vi "harmonics_2021a.vi"() -> ()   [LabVIEW 2024]
uses:
  <vilib>/Analysis/5stat.llb/RMS (DBL).vi
  <vilib>/Utility/file.llb/Read Delimited Spreadsheet (DBL).vi
  <vilib>/measure/matone.llb/Harmonic Distortion Analyzer 1 Chan.vi
  <vilib>/measure/matone.llb/Extract Multiple Tone Information 1 Chan.vi
  <vilib>/measure/NI_MAPro.lvlib
  <vilib>/Analysis/NI_AALPro.lvlib
panel:
  out "grafic energieni consumate":dbl[](graph)
  out "timp":dbl
  out "E [Ws]":dbl
  in  "file path (dialog if empty)":path=path "C:/Users/ciprian/OneDrive - Universitatea Politehnica Timisoara/DESKTOP-LAPTOP HOME 12.12.2021/GR 1 _ 2 _PS_2021.txt"
  in  "Nr_spire":dbl=5.0
  out "D [VAD]":dbl
  out "Q [VA]":dbl
  out "P [W]":dbl
  out "S [VA]":dbl
  out "rms value voltage":dbl format="%0.2f"
  out "rms current 3rd harmonic":dbl format="%0.2f"
  out "rms currnt fundamental":dbl format="%0.2f"
  out "3rd harmonic graph":waveform(dbl)(graph)
  out "3rd current harmonic signal":waveform(dbl)
  in  "export mode 2":T1(ring)=enum."harmonics only"
  in  "export mode":T1(ring)=enum."fundamental signal"
  out "fundamental signal":waveform(dbl)
  out "fundamental graph":waveform(dbl)(graph)
  out "multiple tone information":T2(array[cluster]) {"detected phase (deg)" format="%_6g"; "detected amplitude" format="%_6p"; "detected frequency" format="%_6p"}
  out "input signal graph":dbl[](graph)
  out "t          UMv       UMi           E":dbl[][](array[numeric])
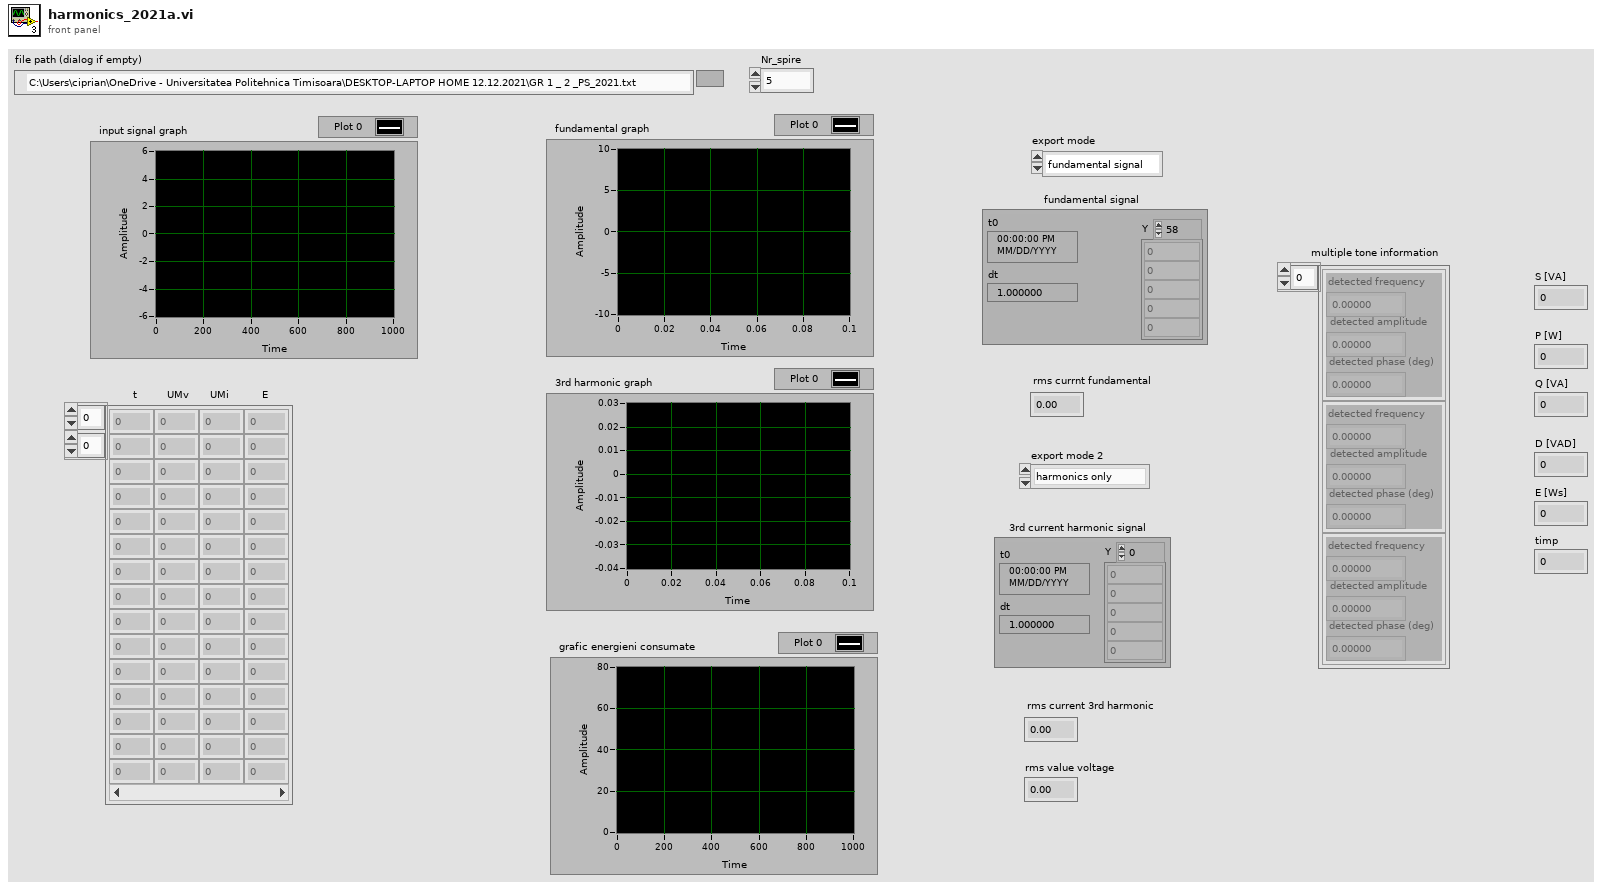
[diagram p1: front panel]
types:
  T1 = enum16{"none", "input signal", "fundamental signal", "residual signal", "harmonics only", "noise and spurs"}
  T2 = cluster{"detected frequency":dbl, "detected amplitude":dbl, "detected phase (deg)":dbl}[]
  T3 = enum32{"none", "input signal", "detected signal", "residual signal"}
  T4 = cluster{"exported time signal":waveform(dbl), "exported spectrum (dB)":cluster{"f0":dbl, "df":dbl, "dB Spectrum (Hann)":dbl[]}}
  T5 = cluster{"detected frequency":dbl, "detected amplitude":dbl, "detected phase (deg)":dbl}
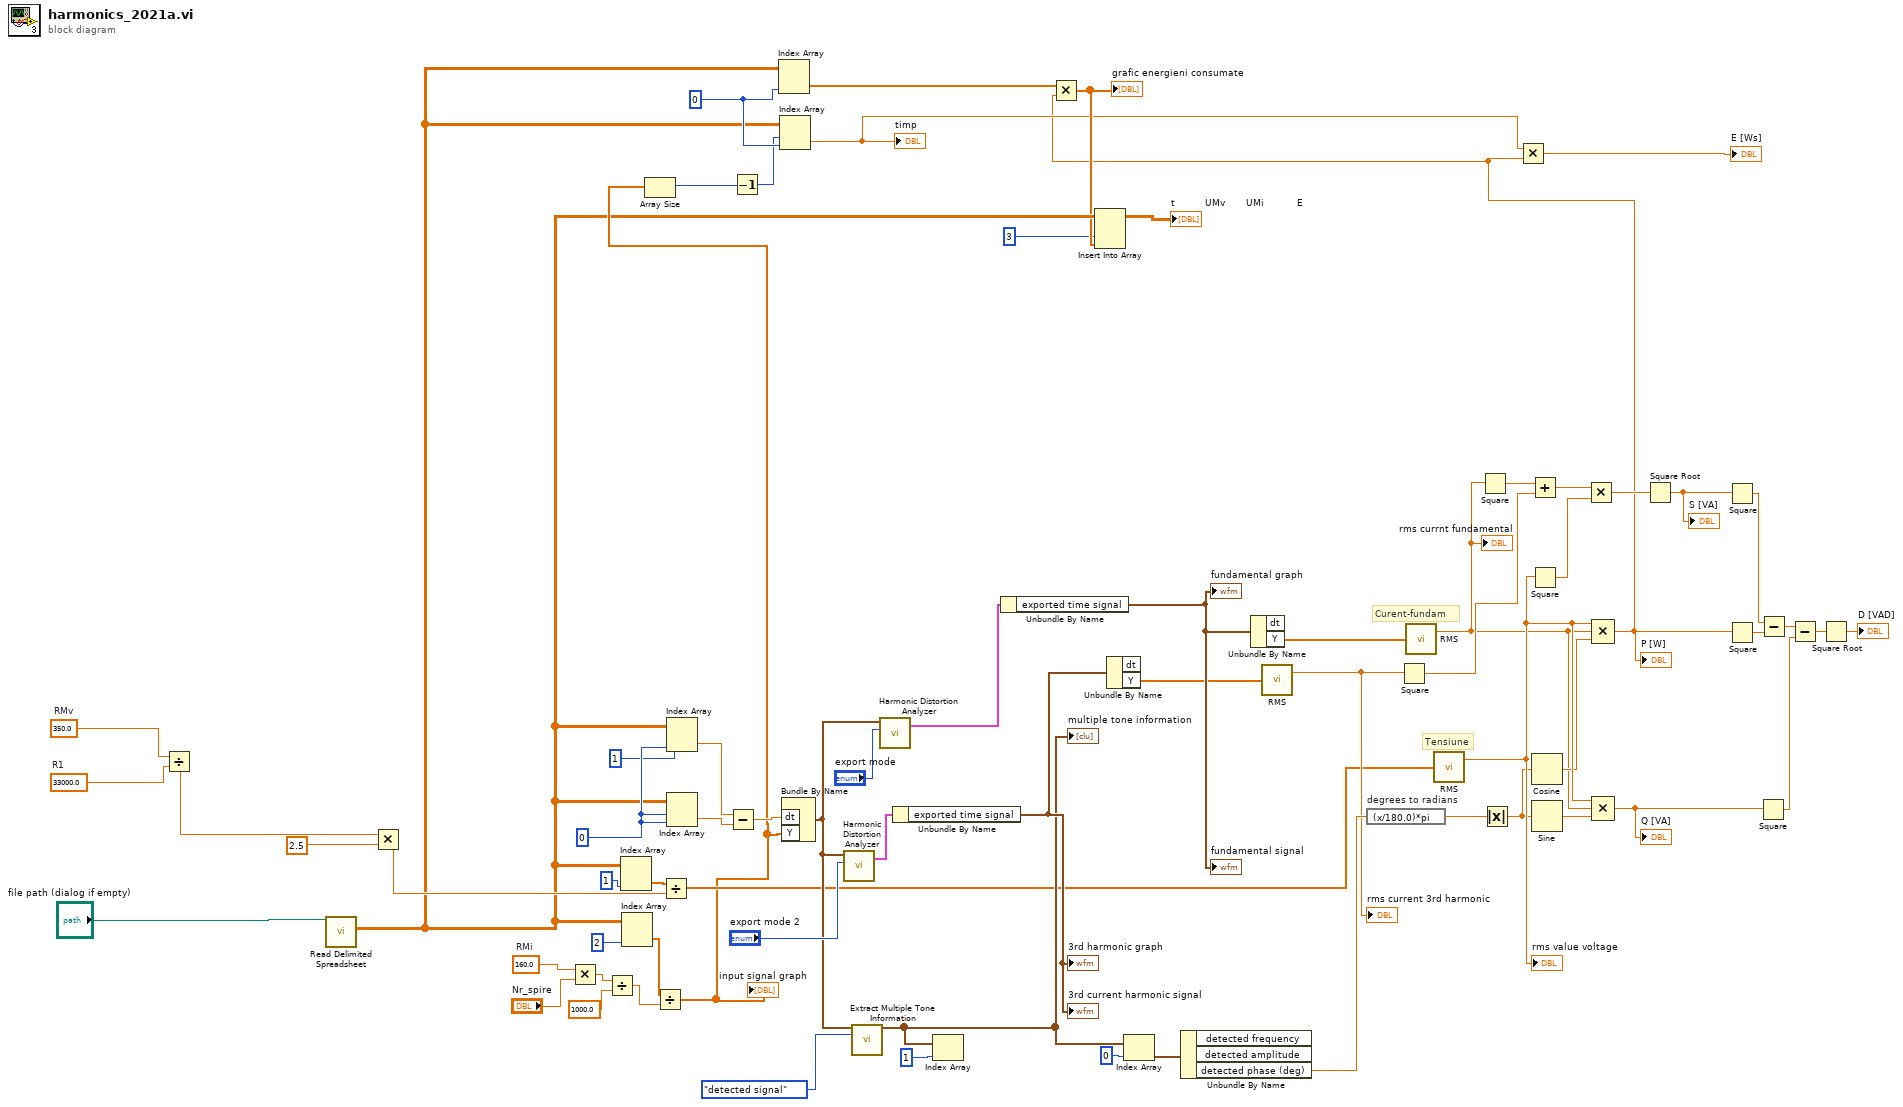
[diagram p0: block diagram]
diagram:
  w12 = 0 ("index (row)")
  w18 = 350.0  # RMv
  w17 = 33000.0  # R1
  w26 = 160.0  # RMi
  w58 = 0 ("index (row)")
  # "Curent-fundam"
  # "Tensiune"
  n1 = Divide(x=w18, y=w17) -> (x/y=w16:dbl)
  n2 = call-poly <vilib>:"Read Delimited Spreadsheet.vi"("file path (dialog if empty)"="file path (dialog if empty)") -> ("all rows"=w7:dbl[][])  [unwired: 9 in, 5 out]
  n3 = Multiply(x=w16, y=2.5) -> (x*y=w14:dbl)
  n4 = Multiply(x=w26, y="Nr_spire") -> (x*y=w24:dbl)
  n5 = Divide(x=w24, y=1000.0) -> (x/y=w22:dbl)
  n6 = Index Array "Index Array"(array=w7, index (col)=1 ("disabled index (col)")) -> (element=w20:dbl[])  [unwired: 1 in]
  n7 = Index Array "Index Array"(array=w7, index (col)=2 ("disabled index (col)")) -> (element=w21:dbl[])  [unwired: 1 in]
  n8 = Divide(x=w21, y=w22) -> (x/y=w9:dbl[])
  "input signal graph" <- w9
  n9 = Array Size(array=w9) -> (size(s)=w10:i32)
  n10 = Divide(x=w20, y=w14) -> (x/y=w19:dbl[])
  n11 = Index Array "Index Array"(array=w7, index (row)=1, index (col)=w58) -> (element=w65:dbl)
  n12 = Index Array "Index Array"(array=w7, index (row)=w58, index (col)=w58) -> (element=w64:dbl)
  n13 = Subtract(x=w65, y=w64) -> (x-y=w63:dbl)
  n14 = Decrement(x=w10) -> (x-1=w11:i32)
  n15 = Index Array "Index Array"(array=w7, index (col)=w12) -> (element=w8:dbl[])  [unwired: 1 in]
  n16 = Index Array "Index Array"(array=w7, index (row)=w11, index (col)=w12) -> (element=w2:dbl)
  "timp" <- w2
  n17 = Bundle By Name("dt"=w63, "Y"=w9) -> (w60:waveform(dbl))  [unwired: 1 in]
  n18 = call-poly <vilib>:"Harmonic Distortion Analyzer.vi"("export mode"="export mode 2", "signal in"=w60) -> ("exported signals"=w59:T4)  [unwired: 4 in, 5 out]
  n19 = call-poly <vilib>:"Extract Multiple Tone Information.vi"("time signal in"=w60, "export mode"=T3."detected signal") -> ("multiple tone information"=w49:T2)  [unwired: 11 in, 2 out]
  "multiple tone information" <- w49
  n20 = call-poly <vilib>:"Harmonic Distortion Analyzer.vi"("export mode"="export mode", "signal in"=w60) -> ("exported signals"=w66:T4)  [unwired: 4 in, 5 out]
  n21 = Unbundle By Name(w59) -> ("exported time signal"=w53:waveform(dbl))
  "3rd harmonic graph" <- w53
  "3rd current harmonic signal" <- w53
  n22 = Index Array(array=w49, index=1) -> ()  [unwired: 1 out]
  n23 = Unbundle By Name(w66) -> ("exported time signal"=w56:waveform(dbl))
  "fundamental graph" <- w56
  "fundamental signal" <- w56
  n24 = Unbundle By Name(w53) -> ("Y"=w54:dbl[])  [unwired: 1 out]
  n25 = Index Array(array=w49, index=0) -> (element=w48:T5)
  n26 = Unbundle By Name(w48) -> ("detected phase (deg)"=w47:dbl)  [unwired: 2 out]
  n27 = Unbundle By Name(w56) -> ("Y"=w55:dbl[])  [unwired: 1 out]
  n28 = call-poly <vilib>:"RMS.vi"("X"=w54) -> ("rms value"=w35:dbl)  [unwired: 1 out]
  "rms current 3rd harmonic" <- w35
  n29 = expression code="(x/180.0)*pi" "degrees to radians"(w47) -> (w37:dbl)
  n30 = Square(x=w35) -> (x^2=w45:dbl)
  n31 = call-poly <vilib>:"RMS.vi"("X"=w55) -> ("rms value"=w38:dbl)  [unwired: 1 out]
  "rms currnt fundamental" <- w38
  n32 = call-poly <vilib>:"RMS.vi"("X"=w19) -> ("rms value"=w41:dbl)  [unwired: 1 out]
  "rms value voltage" <- w41
  n33 = Square(x=w38) -> (x^2=w46:dbl)
  n34 = Absolute Value(x=w37) -> (abs(x)=w36:dbl)
  n35 = Add(x=w46, y=w45) -> (x+y=w44:dbl)
  n36 = Square(x=w41) -> (x^2=w43:dbl)
  n37 = Cosine(x=w36) -> (cos(x)=w39:dbl)
  n38 = Sine(x=w36) -> (sin(x)=w40:dbl)
  n39 = Multiply(x=w44, y=w43) -> (x*y=w42:dbl)
  n40 = Compound Arithmetic op=MULTIPLY(w41, w38, w39) -> (w1:dbl)
  "P [W]" <- w1
  n41 = Multiply(x=w8, y=w1) -> (x*y=w5:dbl[])
  "grafic energieni consumate" <- w5
  n42 = Insert Into Array "Insert Into Array"(array=w7, index (col)=3 ("index (row)"), new element=w5) -> (→"t          UMv       UMi           E":dbl[][])  [unwired: 1 in]
  n43 = Multiply(x=w2, y=w1) -> (x*y=→"E [Ws]":dbl)
  n44 = Compound Arithmetic op=MULTIPLY(w41, w38, w40) -> (w33:dbl)
  "Q [VA]" <- w33
  n45 = Square Root(x=w42) -> (sqrt(x)=w34:dbl)
  "S [VA]" <- w34
  n46 = Square(x=w34) -> (x^2=w32:dbl)
  n47 = Square(x=w1) -> (x^2=w31:dbl)
  n48 = Square(x=w33) -> (x^2=w29:dbl)
  n49 = Subtract(x=w32, y=w31) -> (x-y=w30:dbl)
  n50 = Subtract(x=w30, y=w29) -> (x-y=w28:dbl)
  n51 = Square Root(x=w28) -> (sqrt(x)=→"D [VAD]":dbl)
